vi "Update Control.vi"(8 "error in (no error)":errorcluster, 10 "Updated Controls":refnum<class "Object.lvclass">[](array[class]), 11 "Cluster in":refnum<class "Cluster.lvclass">) -> (0 "error out":errorcluster, 3 "Cluster out":refnum<class "Cluster.lvclass">)   [LabVIEW 2017, in "Front Panel Publisher.lvlib" / "Cluster.lvclass"]
uses:
  Cluster.lvclass
  Object_class/Object.lvclass
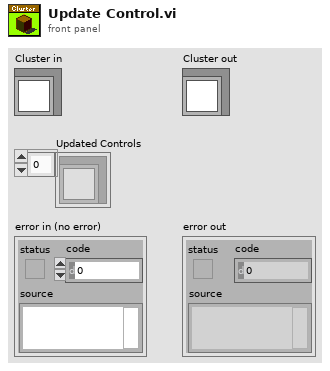
[diagram p1: front panel]
types:
  T1 = typedef "Front Panel Publisher.lvlib/Cluster.lvclass/Attributes.ctl" = cluster{"Cluster Decoration":refnum<class "Object.lvclass">, "Cluster Objects":refnum<class "Object.lvclass">[]}
  T2 = typedef "Front Panel Publisher.lvlib/Object.lvclass/Attributes.ctl" = cluster{"UID":i32, "Type":string, "Starting Location":T3, "Reference":refnum<vi>, "Cluster Component":bool, "Starting Rect Position":cluster{"Left":i16, "Top":i16}, "Owning Pane":refnum<vi>, "Master Total Rect Delta":T4}
  T3 = typedef "Front Panel Publisher.lvlib/Object.lvclass/Coordinates.ctl" = cluster{"Left":i32, "Top":i32, "Height":u32, "Width":u32}
  T4 = typedef "LVRectTypeDef.ctl" = cluster{"Left":i16, "Top":i16, "Right":i16, "Bottom":i16}
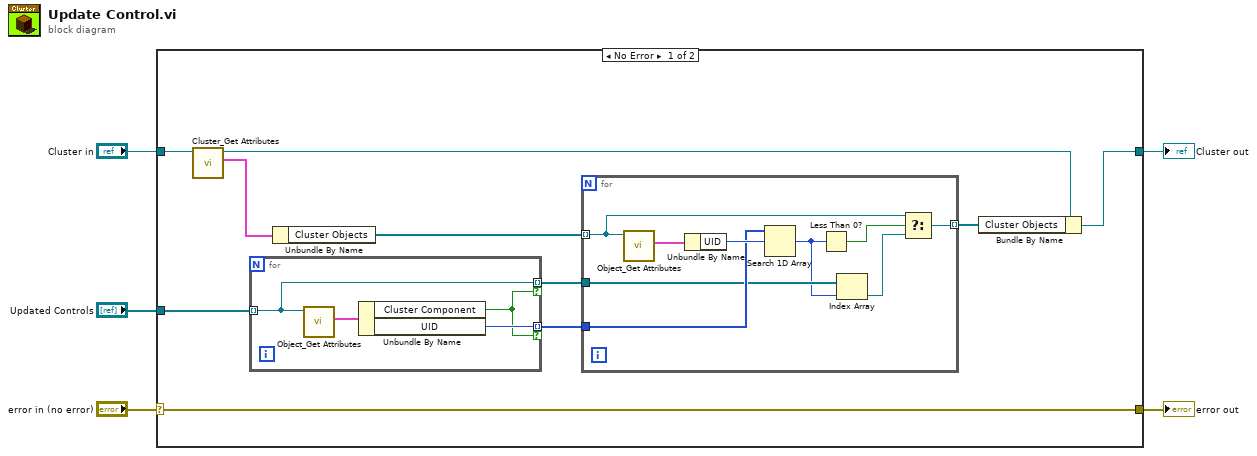
[diagram p0: block diagram]
diagram:
  n1 = case shown="No Error" "error in (no error)" {
    selector: "error in (no error)" -> [w15 w30]
    tunnel: [w15 w30] -> w4
    tunnel: [w6 w29] -> w2
    tunnel: "Cluster in" -> [w14 w29]
    tunnel: "Updated Controls" -> [w11 _]
    frame No Error {
      n2 = call "Cluster_Get Attributes.vi"("Cluster In"=w14) -> ("Cluster Attributes"=w13:T1, "Cluster Out"=w8:refnum<class "Cluster.lvclass">)  [unwired: 8 in, 1 out]
      n3 = for {
        tunnel: w11 -> [w27] mode=indexing
        tunnel: [w27] -> w9 mode=indexing if=w25
        tunnel: [w26] -> w10 mode=indexing if=w25
        n4 = call "Object_Get Attributes.vi"("Object In"=w27) -> ("Object Attributes"=w28:T2)  [unwired: 8 in, 2 out]
        n5 = Unbundle By Name(w28) -> ("Cluster Component"=w25:bool, "UID"=w26:i32)
      }
      n6 = Unbundle By Name(w13) -> ("Cluster Objects"=w12:refnum<class "Object.lvclass">[])
      n7 = for {
        tunnel: w12 -> [w20] mode=indexing
        tunnel: w10 -> [w22]
        tunnel: w9 -> [w19]
        tunnel: [w16] -> w7 mode=indexing
        n8 = call "Object_Get Attributes.vi"("Object In"=w20) -> ("Object Attributes"=w24:T2)  [unwired: 8 in, 2 out]
        n9 = Unbundle By Name(w24) -> ("UID"=w23:i32)
        n10 = Search 1D Array(1D array=w22, element=w23) -> (index of element=w18:i32)  [unwired: 1 in]
        n11 = Less Than 0?(x=w18) -> (x < 0?=w21:bool)
        n12 = Index Array(array=w19, index=w18) -> (element=w17:refnum<class "Object.lvclass">)
        n13 = Select(t=w20, s=w21, f=w17) -> (s? t:f=w16:refnum<class "Object.lvclass">)
      }
      n14 = Bundle By Name(cluster=w8, "Cluster Objects"=w7) -> (w6:refnum<class "Cluster.lvclass">)
    }
    frame Error {
    }
  }
  "error out" <- w4
  "Cluster out" <- w2
